vi "Efficiency+LLR.vi"() -> ()   [LabVIEW 2020]
doc: "Demonstrates how to use triggers and events to synchronize multiple channels in Sequence source mode. Use this example to sequence multiple channels in lock-step."
uses:
  controls/eff_llr_nightwing_config.ctl
  controls/eff_llr_heatwave_config.ctl
  pmbus_ltm4676a/controls/ltm4676a_config.ctl
  controls/eff_llr_system_timing_config.ctl
  <instrlib>/niDCPower/nidcpower.llb/niDCPower Sense.ctl
  <instrlib>/niDCPower/nidcpower.llb/niDCPower Wait For Event - Event.ctl
  <instrlib>/niDCPower/nidcpower.llb/niDCPower Source Mode.ctl
  <instrlib>/niDCPower/nidcpower.llb/niDCPower Output Function.ctl
  <instrlib>/niDCPower/nidcpower.llb/niDCPower Sequence Attribute Type.ctl
  <vilib>/Analysis/1siggen.llb/Ramp Pattern by Samples.vi
  <instrlib>/niDCPower/nidcpower.llb/niDCPower Create Advanced Sequence Step.vi
  <instrlib>/niDCPower/nidcpower.llb/niDCPower Configure Digital Edge Source Trigger.vi
  <instrlib>/niDCPower/nidcpower.llb/niDCPower Configure Digital Edge Measure Trigger.vi
  <vilib>/Utility/file.llb/Write Delimited Spreadsheet (string).vi
  <vilib>/Utility/file.llb/Write Delimited Spreadsheet (DBL).vi
  <vilib>/Analysis/NI_AALBase.lvlib
panel:
  in  "App control":enum32{"Main", "Info", "Ref", "Debug"}(tab)
  out "Test time (s)":dbl
  in  "Config control":T1(tab)
  in  "Source config":T2={"Source device name"="PXIe-4151", "Source device channel"="0", "Source current limit (A)"=25.0, "Source power boundary (W)"=300.0, "Source values (V)"=[9.0, 12.0, 18.0, 20.0]}
  in  "Load config":T3={"Load device name"="PXIe-4051", "Load device channel"="0", "Load voltage limit (V)"=6.0, "Sweep type"=1, "Points or Points/Decade"=10, "Current load level start"=0.1, "Current load level stop"=24.0} {"Current load level stop" min=0.0 step=0.1; "Current load level start" min=0.0 step=0.1; "Points or Points/Decade" min=1; "Sweep type" items=["Linear", "Logarithmic"]}
  in  "System timing config":T4={"DUT setup time (s)"=1.0, "Source delay (s)"=0.005, "Aperture time (s)"=0.005, "Timeout (s)"=15.0} {"Timeout (s)" format="%.3p"; "DUT setup time (s)" format="%.2p"}
  in  "LTM4676A Runtime Config":T5={"SDC config path"=path "C:/dev/users/qkocian/opp_support/demos/argus-buck-demo/instrumentstudio/sdc/pmbus_ltm4676a.sdconfig", "Output setpoint (V)"=3.3, "Voltage margin (%)"=5.0, "Voltage warn limit (%)"=7.5, "Voltage fault limit (%)"=10.0, "Switching frequency (kHz)"=650} {"Switching frequency (kHz)" items=["250"=62440, "350"=64188, "425"=64338, "500"=64488, "575"=575, "650"=650, "750"=750, "1000"=1000]; "Voltage fault limit (%)" min=0.0 max=100.0 step=1.0 format="%.1g"; "Voltage warn limit (%)" min=0.0 max=100.0 step=1.0 format="%.1g"; "Voltage margin (%)" min=0.0 max=100.0 step=1.0 format="%.1g"; "Output setpoint (V)" min=0.5 max=5.5 step=0.1}
  out "Load Current (A) vs DUT Output Voltage (V)":T6(graph) caption="Current (Amps) vs Voltage (Volts)"
  out "DUT Efficiency (%) vs. Load Current (A)":cluster{dbl[], dbl[]}[](graph) caption="Current (Amps) vs Voltage (Volts)"
  in  "Use PMBus?":bool
  out "success?":bool
  in  "Export debug curves?":enum16{"No", "Yes"}(ring)
  out "Load Power":T7(graph) caption="Current (Amps) vs Voltage (Volts)"
  out "Supply Power":T7(graph) caption="Current (Amps) vs Voltage (Volts)"
  out "Load Current":T7(graph) caption="Current (Amps) vs Voltage (Volts)"
  out "Load Voltage":cluster{dbl[], "voltage measurements":dbl[]}(graph) caption="Current (Amps) vs Voltage (Volts)"
  out "Supply Current":T7(graph) caption="Current (Amps) vs Voltage (Volts)"
  out "Supply Voltage":T8(graph) caption="Current (Amps) vs Voltage (Volts)"
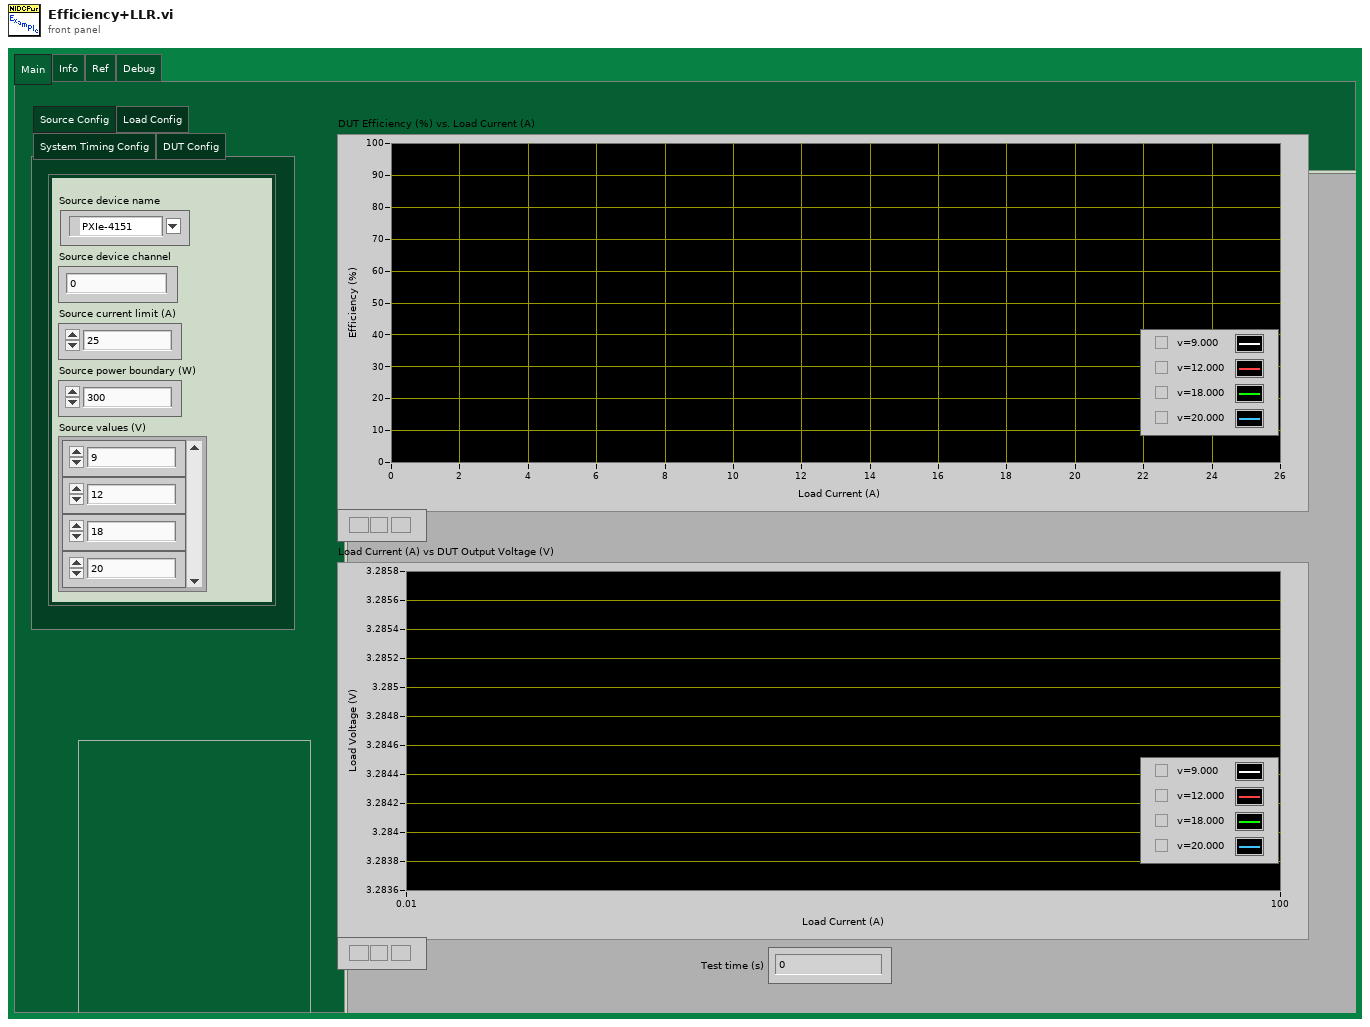
[diagram p1: front panel]
types:
  T1 = enum32{"Source Config", "Load Config", "System Timing Config", "DUT Config"}
  T2 = typedef "eff_llr_nightwing_config.ctl" = cluster{"Source device name":refnum<k15>, "Source device channel":string, "Source current limit (A)":dbl, "Source power boundary (W)":dbl, "Source values (V)":dbl[]}
  T3 = typedef "eff_llr_heatwave_config.ctl" = cluster{"Load device name":refnum<k15>, "Load device channel":string, "Load voltage limit (V)":dbl, "Sweep type":u16, "Points or Points/Decade":i32, "Current load level start":dbl, "Current load level stop":dbl}
  T4 = typedef "eff_llr_system_timing_config.ctl" = cluster{"DUT setup time (s)":dbl, "Source delay (s)":dbl, "Aperture time (s)":dbl, "Timeout (s)":dbl}
  T5 = typedef "ltm4676a_config.ctl" = cluster{"SDC config path":path, "Output setpoint (V)":dbl, "Voltage margin (%)":dbl, "Voltage warn limit (%)":dbl, "Voltage fault limit (%)":dbl, "Switching frequency (kHz)":u16}
  T6 = cluster{"current measurements":dbl[], "voltage measurements":dbl[]}[]
  T7 = cluster{"Ramp Pattern":dbl[], "current measurements":dbl[]}
  T8 = cluster{"Ramp Pattern":dbl[], "voltage measurements":dbl[]}
  T9 = typedef "niDCPower Source Mode.ctl" = i32
  T10 = typedef "niDCPower Wait For Event - Event.ctl" = i32
  T11 = typedef "niDCPower Sense.ctl" = i32
  T12 = typedef "niDCPower Sequence Attribute Type.ctl" = i32
  T13 = typedef "niDCPower Output Function.ctl" = i32
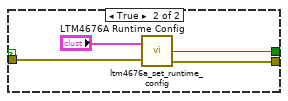
[diagram p2: hidden frame]
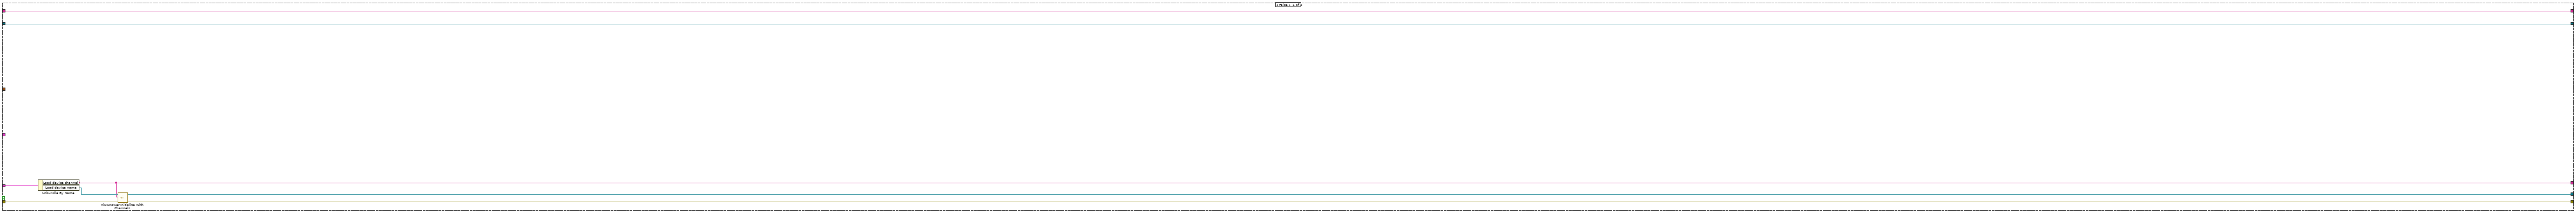
[diagram p3: hidden frame]
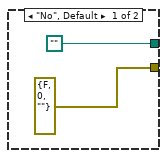
[diagram p5: hidden frame]
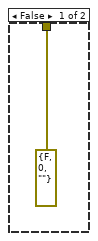
[diagram p6: hidden frame]
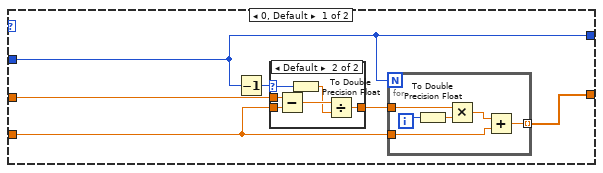
[diagram p7: hidden frame]
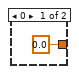
[diagram p8: hidden frame]
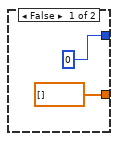
[diagram p9: hidden frame]
diagram:
  w25 = 1038 items=["Slow"=1041, "Normal"=1038, "Fast"=1039, "Custom"=1042] ("Source:Transient Response")
  w35 = T9 1020 items=["Single Point"=1020, "Sequence"=1021] ("source mode")
  w40 = 1006 items=["DC Voltage"=1006, "DC Current"=1007, "Pulse Voltage"=1049, "Pulse Current"=1050] ("Source:Output Function")
  w47 = T10 1030 items=["Source Complete Event"=1030, "Measure Complete Event"=1031, "Sequence Iteration Complete Event"=1032, "Sequence Engine Done Event"=1033, "Pulse Complete Event"=1051, "Ready For Pulse Trigger Event"=1052] ("event")
  w50 = 1 items=["Off", "On"] ("Source:DC Current:Current Level Autorange")
  w53 = T11 1009 items=["Local"=1008, "Remote"=1009] ("sense")
  n1 = Unbundle By Name("Source config") -> ("Source device channel"=w14:string, "Source device name"=w18:refnum<k15>)
  n2 = call <instrlib>:"niDCPower Initialize With Channels.vi"("channels"=w14, "resource name"=w18) -> ("error out"=w51:errorcluster, "instrument handle out"=w52:refnum<k15>)  [unwired: 3 in, 5 out]
  n3 = Unbundle By Name("System timing config") -> ("DUT setup time (s)"=w20:dbl)
  n4 = Unbundle By Name("Source config") -> ("Source values (V)"=w15:dbl[], "Source current limit (A)"=w17:dbl)
  n5 = call <instrlib>:"niDCPower Configure Sense.vi"("error in (no error)"=w51, "sense"=w53, "channel name"=w14, "instrument handle"=w52) -> ("error out"=w37:errorcluster, "instrument handle out"=w39:refnum<k15>)  [unwired: 6 in]
  n6 = call <instrlib>:"niDCPower Configure Source Mode With Channels.vi"("error in (no error)"=w37, "source mode"=w35, "channel name"=w14, "instrument handle"=w39) -> ("error out"=w36:errorcluster, "instrument handle out"=w38:refnum<k15>)  [unwired: 6 in]
  n7 = Index Array(array=w15, index=0) -> (element=w42:dbl)
  n8 = property class="niDCPower"(reference=w38, error in=w36, "Active Channel"=w14, "Output Function"=w40, "Voltage Level"=w42, "Current Limit"=w17, "Voltage Level Autorange"=w50, "Current Limit Autorange"=w50, "Source Delay"=w20) -> (reference out=w27:refnum<k15>, error out=w26:errorcluster)
  n9 = property class="niDCPower"(reference=w27, error in=w26, "Active Channel"=w14, "Transient Response"=w25) -> (reference out=w23:refnum<k15>, error out=w24:errorcluster)
  n10 = call <instrlib>:"niDCPower Commit With Channels.vi"("error in (no error)"=w24, "channel name"=w14, "instrument handle"=w23) -> ("error out"=w21:errorcluster, "instrument handle out"=w22:refnum<k15>)  [unwired: 7 in]
  n11 = call <instrlib>:"niDCPower Initiate With Channels.vi"("error in (no error)"=w21, "channel name"=w14, "instrument handle"=w22) -> ("error out"=w49:errorcluster, "instrument handle out"=w48:refnum<k15>)  [unwired: 7 in]
  n12 = call <instrlib>:"niDCPower Wait For Event With Channels.vi"("error in (no error)"=w49, "event"=w47, "channel name"=w14, "instrument handle"=w48) -> ("error out"=w46:errorcluster, "instrument handle out"=w45:refnum<k15>)  [unwired: 6 in]
  n13 = call <instrlib>:"niDCPower Measure Multiple.vi"("error in (no error)"=w46, "channel name"=w14, "instrument handle"=w45) -> ("error out"=w43:errorcluster, "instrument handle out"=w44:refnum<k15>)  [unwired: 5 in, 2 out]
  n14 = call <instrlib>:"niDCPower Abort With Channels.vi"("error in (no error)"=w43, "channel name"=w14, "instrument handle"=w44) -> ("error out"=w13:errorcluster, "instrument handle out"=w41:refnum<k15>)  [unwired: 7 in]
  n15 = case shown="False" "Use PMBus?" {
    tunnel: w13 -> [w59 w63]
    tunnel: [w59 w61] -> w12
    tunnel: [TRUE ("success?") w60] -> w4
    frame False {
    }
    frame True {
      n16 = call "ltm4676a_set_runtime_config.vi"("LTM4676A Runtime Config"="LTM4676A Runtime Config", "error in (no error)"=w63) -> ("success?"=w60:bool, "error out"=w61:errorcluster)  [unwired: 1 out]
    }
  }
  "success?" <- w4
  n17 = call <vilib>:"High Resolution Relative Seconds.vi"() -> ("relative seconds"=w2:dbl)
  n18 = case shown="True" w4 {
    tunnel: w41 -> [w68 w141]
    tunnel: [w64 w129] -> w28
    tunnel: "System timing config" -> [_ w104]
    tunnel: "Source config" -> [_ w98]
    tunnel: w14 -> [w69 w94]
    tunnel: w12 -> [w66 w88]
    tunnel: [w66 w84] -> w9
    tunnel: [w68 w83] -> w7
    tunnel: [w69 w82] -> w6
    tunnel: [w65 w81] -> w5
    tunnel: "Load config" -> [w67 w73]
    tunnel: w2 -> [_ w72]
    frame False {
      n19 = Unbundle By Name(w67) -> ("Load device channel"=w64:string, "Load device name"=w65:refnum<k15>)
      n20 = call <instrlib>:"niDCPower Initialize With Channels.vi"("error in (no error)"=w66, "channels"=w64, "resource name"=w65) -> ()  [unwired: 2 in, 7 out]
    }
    frame True {
      w119 = 1038 items=["Slow"=1041, "Normal"=1038, "Fast"=1039, "Custom"=1042] ("Source:Transient Response")
      w131 = T9 1020 items=["Single Point"=1020, "Sequence"=1021] ("source mode")
      w148 = T10 1030 items=["Source Complete Event"=1030, "Measure Complete Event"=1031, "Sequence Iteration Complete Event"=1032, "Sequence Engine Done Event"=1033, "Pulse Complete Event"=1051, "Ready For Pulse Trigger Event"=1052] ("event")
      w153 = 1 items=["Off", "On"] ("Source:DC Current:Current Level Autorange")
      w154 = 1007 items=["DC Voltage"=1006, "DC Current"=1007, "Pulse Voltage"=1049, "Pulse Current"=1050] ("Source:Output Function")
      w173 = T11 1009 items=["Local"=1008, "Remote"=1009] ("sense")
      w178 = 1 items=["Off", "On"] ("DC Voltage:Voltage Level Autorange")
      w179 = T12[] [1250001, 1250005] items=["Source -> Output Function"=1150008, "Source -> Output Enabled"=1250006, "Source -> Output Resistance"=1150061, "Source -> Transient Response"=1150062, "Source -> Custom Transient Response -> Voltage Gain Bandwidth"=1150067, "Source -> Custom Transient Response -> Voltage Compensation Frequency"=1150068, "Source -> Custom Transient Response -> Voltage Pole-Zero Ratio"=1150069, "Source -> Custom Transient Response -> Current Gain Bandwidth"=1150070, "Source -> Custom Transient Response -> Current Compensation Frequency"=1150071, "Source -> Custom Transient Response -> Current Pole-Zero Ratio"=1150072, "Source -> DC Voltage -> Voltage Level"=1250001, "Source -> DC Voltage -> Voltage Level Range"=1150005, "Source -> DC Voltage -> Current Limit"=1250005, "Source -> DC Voltage -> Current Limit High"=1150187, "Source -> DC Voltage -> Current Limit Low"=1150188, "Source -> DC Voltage -> Current Limit Range"=1150004, "Source -> DC Current -> Current Level"=1150009, "Source -> DC Current -> Current Level Range"=1150011, "Source -> DC Current -> Voltage Limit"=1150010, "Source -> DC Current -> Voltage Limit High"=1150185, "Source -> DC Current -> Voltage Limit Low"=1150186, "Source -> DC Current -> Voltage Limit Range"=1150012, "Source -> Pulse Voltage -> Pulse Voltage Level"=1150080, "Source -> Pulse Voltage -> Pulse Bias Voltage Level"=1150082, "Source -> Pulse Voltage -> Pulse Voltage Level Range"=1150084, "Source -> Pulse Voltage -> Pulse Current Limit"=1150081, "Source -> Pulse Voltage -> Pulse Current Limit High"=1150193, "Source -> Pulse Voltage -> Pulse Current Limit Low"=1150194, "Source -> Pulse Voltage -> Pulse Bias Current Limit"=1150083, "Source -> Pulse Voltage -> Pulse Bias Current Limit High"=1150195, "Source -> Pulse Voltage -> Pulse Bias Current Limit Low"=1150196, "Source -> Pulse Voltage -> Pulse Current Limit Range"=1150085, "Source -> Pulse Current -> Pulse Current Level"=1150086, "Source -> Pulse Current -> Pulse Bias Current Level"=1150088, "Source -> Pulse Current -> Pulse Current Level Range"=1150090, "Source -> Pulse Current -> Pulse Voltage Limit"=1150087, "Source -> Pulse Current -> Pulse Voltage Limit High"=1150189, "Source -> Pulse Current -> Pulse Voltage Limit Low"=1150190, "Source -> Pulse Current -> Pulse Bias Voltage Limit"=1150089, "Source -> Pulse Current -> Pulse Bias Voltage Limit High"=1150191, "Source -> Pulse Current -> Pulse Bias Voltage Limit Low"=1150192, "Source -> Pulse Current -> Pulse Voltage Limit Range"=1150091, "Source -> Advanced -> Source Delay"=1150051, "Source -> Advanced -> Pulse Bias Delay"=1150092, "Source -> Advanced -> Pulse On Time"=1150093, "Source -> Advanced -> Pulse Off Time"=1150094, "Source -> Advanced -> OVP Enabled"=1250002, "Source -> Advanced -> OVP Limit"=1250003, "Source -> Advanced -> Compliance Limit Symmetry"=1150184, "Source -> Advanced -> Sequence Step Delta Time"=1150198, "Measurement -> Sense"=1150013, "Measurement -> Aperture Time"=1150058, "Measurement -> Measure Record Length"=1150063, "Measurement -> Advanced -> DC Noise Rejection"=1150066, "Measurement -> Autorange"=1150244, "Measurement -> Advanced -> Autorange Behavior"=1150245, "Measurement -> Advanced -> Autorange Aperture Time Mode"=1150246, "Measurement -> Advanced -> Autorange Minimum Aperture Time"=1150247, "Measurement -> Advanced -> Autorange Minimum Aperture Time Units"=1150248, "Measurement -> Advanced -> Autorange Minimum Current Range"=1150255, "Measurement -> Advanced -> Autorange Minimum Voltage Range"=1150256, "Measurement -> Advanced -> Autorange Threshold Mode"=1150257, "Measurement -> Advanced -> Autorange Maximum Delay After Range Change"=1150322, "LCR -> Instrument Mode"=1150208, "LCR -> LCR Stimulus Function"=1150209, "LCR -> LCR Frequency"=1150210, "LCR -> LCR Voltage Amplitude"=1150211, "LCR -> LCR Current Amplitude"=1150212, "LCR -> LCR DC Bias Source"=1150213, "LCR -> LCR DC Bias Voltage Level"=1150214, "LCR -> LCR DC Bias Current Level"=1150215, "LCR -> LCR Impedance Autorange"=1150216, "LCR -> LCR Impedance Range"=1150217, "LCR -> LCR Measurement Time"=1150218, "LCR -> LCR Custom Measurement Time"=1150258, "LCR -> LCR Source Delay Mode"=1150315, "LCR -> Compensation -> Open -> Enabled"=1150220, "LCR -> Compensation -> Open -> Conductance"=1150261, "LCR -> Compensation -> Open -> Susceptance"=1150262, "LCR -> Compensation -> Short -> Enabled"=1150221, "LCR -> Compensation -> Short -> Resistance"=1150263, "LCR -> Compensation -> Short -> Reactance"=1150264, "LCR -> Compensation -> Load -> Enabled"=1150222, "LCR -> Compensation -> Load -> Measured Resistance"=1150268, "LCR -> Compensation -> Load -> Measured Reactance"=1150269, "LCR -> Compensation -> Load -> Actual Resistance"=1150270, "LCR -> Compensation -> Load -> Actual Reactance"=1150271] ("advanced sequence properties")
      w112 = "SourceVoltages" ("sequence name")
      w182 = T13 1007 items=["DC Voltage"=1006, "DC Current"=1007, "Pulse Voltage"=1049, "Pulse Current"=1050] ("output function")
      w183 = 1027 items=["Automatically after Source Complete"=1025, "On Demand"=1026, "On Measure Trigger"=1027] ("Measurement:Advanced:Measure When")
      w184 = T9 1021 items=["Single Point"=1020, "Sequence"=1021] ("source mode")
      w191 = T13 1006 items=["DC Voltage"=1006, "DC Current"=1007, "Pulse Voltage"=1049, "Pulse Current"=1050] ("output function")
      w128 = 1025 items=["Automatically after Source Complete"=1025, "On Demand"=1026, "On Measure Trigger"=1027] ("Measurement:Advanced:Measure When")
      w198 = T9 1021 items=["Single Point"=1020, "Sequence"=1021] ("source mode")
      n21 = Unbundle By Name(w73) -> ("Load device channel"=w75:string, "Load device name"=w74:refnum<k15>)
      n22 = Unbundle By Name(w73) -> ("Load voltage limit (V)"=w80:dbl, "Sweep type"=w79:u16, "Points or Points/Decade"=w78:i32, "Current load level stop"=w77:dbl, "Current load level start"=w76:dbl)
      n23 = local read "System timing config"() -> (w109:T4)
      n24 = call <instrlib>:"niDCPower Initialize With Channels.vi"("error in (no error)"=w88, "channels"=w75, "resource name"=w74) -> ("error out"=w151:errorcluster, "instrument handle out"=w152:refnum<k15>)  [unwired: 2 in, 5 out]
      n25 = Unbundle By Name(w109) -> ("DUT setup time (s)"=w108:dbl)
      n26 = call <instrlib>:"niDCPower Configure Sense.vi"("error in (no error)"=w151, "sense"=w173, "channel name"=w75, "instrument handle"=w152) -> ("error out"=w134:errorcluster, "instrument handle out"=w135:refnum<k15>)  [unwired: 6 in]
      n27 = call <instrlib>:"niDCPower Configure Source Mode With Channels.vi"("error in (no error)"=w134, "source mode"=w131, "channel name"=w75, "instrument handle"=w135) -> ("error out"=w132:errorcluster, "instrument handle out"=w133:refnum<k15>)  [unwired: 6 in]
      n28 = case shown="1" w79 {
        tunnel: w78 -> [w327 w346]
        tunnel: [w330 w350] -> w175
        tunnel: w76 -> [w329 w347]
        tunnel: w77 -> [w328 w354]
        tunnel: [w327 w351] -> w168
        frame 0, Default {
          n29 = Decrement(x=w327) -> (x-1=w332:i32)
          n30 = case shown="Default" w332 {
            selector: w332 -> [_ w340]
            tunnel: w328 -> [_ w345]
            tunnel: w329 -> [_ w344]
            tunnel: [0.0 w342] -> w331
            frame 0 {
            }
            frame Default {
              n31 = Subtract(x=w345, y=w344) -> (x-y=w343:dbl)
              n32 = To Double Precision Float(number=w340) -> (double precision float=w341:dbl)
              n33 = Divide(x=w343, y=w341) -> (x/y=w342:dbl)
            }
          }
          n34 = for {
            N: w327 -> [_]
            tunnel: w331 -> [w337]
            tunnel: w329 -> [w338]
            tunnel: [w333] -> w330 mode=indexing
            i -> [w336]
            n35 = To Double Precision Float(number=w336) -> (double precision float=w334:dbl)
            n36 = Multiply(x=w337, y=w334) -> (x*y=w335:dbl)
            n37 = Add(x=w335, y=w338) -> (x+y=w333:dbl)
          }
        }
        frame 1 {
          n38 = Divide(x=w354, y=w347) -> (x/y=w355:dbl)
          n39 = Logarithm Base 10(1:w355) -> (0:w352:dbl)
          n40 = In Range and Coerce(upper limit=inf, x=w352, lower limit=0.0) -> (In Range?=w349:bool)  [unwired: 1 out]
          n41 = case shown="True" w349 {
            tunnel: [dbl[] [] w365] -> w350
            tunnel: [0 w358] -> w351
            tunnel: w354 -> [_ w364]
            tunnel: w347 -> [_ w363]
            tunnel: w346 -> [_ w360]
            frame False {
            }
            frame True {
              n42 = Reciprocal(x=w360) -> (1/x=w362:dbl)
              n43 = Power Of 10(x=w362) -> (10^x=w361:dbl)
              n44 = while {
                tunnel: w361 -> [w370]
                tunnel: w363 -> [w373]
                tunnel: [w369] -> w365 mode=indexing
                tunnel: [w371] -> w359
                tunnel: w364 -> [w366]
                i -> [w371]
                stop <- w368 continue-if-true
                n45 = Power Of X(1:w370, 2:w371) -> (0:w372:dbl)
                n46 = Multiply(x=w372, y=w373) -> (x*y=w367:dbl)
                n47 = Less?(x=w367, y=w366) -> (x < y?=w368:bool)
                n48 = Select(t=w367, s=w368, f=w366) -> (s? t:f=w369:dbl)
              }
              n49 = Increment(x=w359) -> (x+1=w358:i32)
            }
          }
        }
      }
      n50 = property class="niDCPower"(reference=w133, error in=w132, "Active Channel"=w75, "Output Function"=w154, "Current Level"=1.0 ("Source:DC Current:Current Level"), "Voltage Limit Range"=w80, "Current Level Autorange"=w153, "Source Delay"=w108, "Current Level Range"=40.0 ("Source:DC Current:Current Level Range")) -> (reference out=w121:refnum<k15>, error out=w120:errorcluster)
      n51 = property class="niDCPower"(reference=w121, error in=w120, "Active Channel"=w75, "Transient Response"=w119) -> (reference out=w116:refnum<k15>, error out=w115:errorcluster)
      n52 = Multiply(x=w175, y=1.0) -> (x*y=w163:dbl[])
      n53 = local read "Source config"() -> (w103:T2)
      n54 = call <instrlib>:"niDCPower Commit With Channels.vi"("error in (no error)"=w115, "channel name"=w75, "instrument handle"=w116) -> ("error out"=w118:errorcluster, "instrument handle out"=w117:refnum<k15>)  [unwired: 7 in]
      n55 = call <instrlib>:"niDCPower Initiate With Channels.vi"("error in (no error)"=w118, "channel name"=w75, "instrument handle"=w117) -> ("error out"=w150:errorcluster, "instrument handle out"=w149:refnum<k15>)  [unwired: 7 in]
      n56 = Unbundle By Name(w103) -> ("Source values (V)"=w102:dbl[])
      n57 = call <instrlib>:"niDCPower Wait For Event With Channels.vi"("error in (no error)"=w150, "event"=w148, "channel name"=w75, "instrument handle"=w149) -> ("error out"=w147:errorcluster, "instrument handle out"=w146:refnum<k15>)  [unwired: 6 in]
      n58 = call <instrlib>:"niDCPower Measure Multiple.vi"("error in (no error)"=w147, "channel name"=w75, "instrument handle"=w146) -> ("error out"=w144:errorcluster, "instrument handle out"=w145:refnum<k15>)  [unwired: 5 in, 2 out]
      n59 = Array Size(array=w102) -> (size(s)=w110:i32)
      n60 = call <instrlib>:"niDCPower Abort With Channels.vi"("error in (no error)"=w144, "channel name"=w75, "instrument handle"=w145) -> ("error out"=w139:errorcluster, "instrument handle out"=w140:refnum<k15>)  [unwired: 7 in]
      n61 = for {
        N: w110 -> [_]
        tunnel: w163 -> [w246]
        tunnel: [w245] -> w162 mode=concatenating
        n62 = for {
          tunnel: w246 -> [w247] mode=indexing
          tunnel: [w247] -> w245 mode=indexing
        }
      }
      n63 = call <instrlib>:"niDCPower Configure Source Mode.vi"("error in (no error)"=w139, "source mode"=w198, "instrument handle"=w141) -> ("error out"=w200:errorcluster, "instrument handle out"=w199:refnum<k15>)  [unwired: 7 out]
      n64 = call <instrlib>:"niDCPower Configure Output Function.vi"("error in (no error)"=w200, "output function"=w191, "channel name"=w94, "instrument handle"=w199) -> ("error out"=w142:errorcluster, "instrument handle out"=w143:refnum<k15>)  [unwired: 6 out]
      n65 = property class="niDCPower"(reference=w143, error in=w142, "Active Channel"=w94, "Source:DC Voltage:Voltage Level Autorange"=w178, "Source:DC Voltage:Current Limit Autorange"=w178) -> (reference out=w177:refnum<k15>, error out=w176:errorcluster)
      n66 = Unbundle By Name(w104) -> ("Source delay (s)"=w107:dbl)
      n67 = property class="niDCPower"(reference=w177, error in=w176, "Active Channel"=w94, "Source Delay"=w107) -> (reference out=w91:refnum<k15>, error out=w90:errorcluster)
      n68 = Unbundle By Name(w98) -> ("Source power boundary (W)"=w101:dbl, "Source values (V)"=w100:dbl[], "Source current limit (A)"=w99:dbl)
      n69 = call <instrlib>:"niDCPower Create Advanced Sequence.vi"("instrument handle"=w91, "sequence name"=w112, "advanced sequence properties"=w179, "error in (no error)"=w90) -> ("instrument handle out"=w181:refnum<k15>, "error out"=w180:errorcluster)  [unwired: 10 in]
      n70 = for {
        tunnel: w101 -> [w377]
        tunnel: w99 -> [w376]
        tunnel: w100 -> [w375] mode=indexing
        shift-right: [w379] -> w96
        shift-left: w181 -> [w381]
        shift-right: [w378] -> w95
        shift-left: w180 -> [w380]
        tunnel: w168 -> [w374]
        n71 = for {
          N: w374 -> [_]
          shift-right: [w390] -> w378
          shift-left: w380 -> [w393]
          shift-right: [w389] -> w379
          shift-left: w381 -> [w388]
          tunnel: w377 -> [w387]
          tunnel: w375 -> [w382]
          tunnel: w376 -> [w385]
          n72 = call-poly <instrlib>:"niDCPower Create Advanced Sequence Step (Poly).vi"("error in (no error)"=w393, "instrument handle"=w388) -> ("error out"=w391:errorcluster, "instrument handle out"=w392:refnum<k15>)  [unwired: 8 in]
          n73 = Divide(x=w387, y=w382) -> (x/y=w384:dbl)
          n74 = Less?(x=w384, y=w385) -> (x < y?=w386:bool)
          n75 = Select(t=w384, s=w386, f=w385) -> (s? t:f=w383:dbl)
          n76 = property class="niDCPower"(reference=w392, error in=w391, "Voltage Level"=w382, "Current Limit"=w383) -> (reference out=w389:refnum<k15>, error out=w390:errorcluster)
        }
      }
      n77 = call "buildTerminalName.vi"("error in (no error)"=w95, "Local Terminal Name"="SourceTrigger", "Channel Name"=w94, "session handle"=w96) -> ("error IO"=w92:errorcluster, "Fully Qualified Terminal Name"=w194:string, "session handle 2"=w93:refnum<k15>)  [unwired: 5 out]
      n78 = call "buildTerminalName.vi"("error in (no error)"=w92, "Local Terminal Name"="SourceCompleteEvent", "Channel Name"=w94, "session handle"=w93) -> ("error IO"=w111:errorcluster, "Fully Qualified Terminal Name"=w193:string, "session handle 2"=w127:refnum<k15>)  [unwired: 5 out]
      n79 = Unbundle By Name(w104) -> ("Aperture time (s)"=w106:dbl)
      n80 = property class="niDCPower"(reference=w127, error in=w111, "Measure When"=w128, "Aperture Time"=w106) -> (reference out=w197:refnum<k15>, error out=w196:errorcluster)
      n81 = call <instrlib>:"niDCPower Commit.vi"("error in (no error)"=w196, "instrument handle"=w197) -> ("error out"=w138:errorcluster, "instrument handle out"=w159:refnum<k15>)  [unwired: 8 out]
      n82 = call <instrlib>:"niDCPower Configure Source Mode.vi"("error in (no error)"=w138, "source mode"=w184, "instrument handle"=w140) -> ("error out"=w186:errorcluster, "instrument handle out"=w185:refnum<k15>)  [unwired: 7 out]
      n83 = call <instrlib>:"niDCPower Configure Output Function.vi"("error in (no error)"=w186, "output function"=w182, "instrument handle"=w185) -> ("error out"=w136:errorcluster, "instrument handle out"=w137:refnum<k15>)  [unwired: 1 in, 6 out]
      n84 = call <instrlib>:"niDCPower Set Sequence.vi"("error in (no error)"=w136, "values"=w162, "instrument handle"=w137) -> ("error out"=w164:errorcluster, "instrument handle out"=w165:refnum<k15>)  [unwired: 2 in, 5 out]
      n85 = disable-structure shown="Disabled" {
        disable-tunnel: [w214 w217] -> w172
        disable-tunnel: [w213 w216] -> w171
        disable-tunnel: w165 -> [w212 w217]
        disable-tunnel: w164 -> [w211 w216]
        disable-tunnel: w75 -> [w210 _]
        frame Disabled {
          w215 = 1 items=["Off", "On"] ("DC Voltage:Voltage Level Autorange")
          n86 = property class="niDCPower"(reference=w212, error in=w211, "Active Channel"=w210, "Current Level Autorange"=w215) -> (reference out=w214:refnum<k15>, error out=w213:errorcluster)
        }
        frame Enabled {
        }
      }
      n87 = property class="niDCPower"(reference=w172, error in=w171, "Active Channel"=w75, "Source Delay"=0.0 ("Source:Advanced:Source Delay")) -> (reference out=w167:refnum<k15>, error out=w166:errorcluster)
      n88 = call-poly <instrlib>:"niDCPower Configure Trigger (Poly).vi"("error in (no error)"=w166, "input terminal"=w194, "instrument handle"=w167) -> ("error out"=w189:errorcluster, "instrument handle out"=w190:refnum<k15>)  [unwired: 1 in, 6 out]
      n89 = Unbundle By Name(w104) -> ("Timeout (s)"=w89:dbl, "Aperture time (s)"=w105:dbl)
      n90 = property class="niDCPower"(reference=w190, error in=w189, "Measure When"=w183, "Aperture Time"=w105) -> (reference out=w187:refnum<k15>, error out=w188:errorcluster)
      n91 = call-poly <instrlib>:"niDCPower Configure Trigger (Poly).vi"("error in (no error)"=w188, "input terminal"=w193, "instrument handle"=w187) -> ("error out"=w161:errorcluster, "instrument handle out"=w160:refnum<k15>)  [unwired: 1 in, 6 out]
      n92 = call <instrlib>:"niDCPower Commit.vi"("error in (no error)"=w161, "instrument handle"=w160) -> ("error out"=w201:errorcluster, "instrument handle out"=w202:refnum<k15>)  [unwired: 8 out]
      n93 = flat-sequence {
        tunnel: w202 -> [w225]
        tunnel: w201 -> [w224]
        tunnel: w159 -> [w221]
        tunnel: [w222] -> w209
        tunnel: [w220] -> w208
        tunnel: [w219] -> w207
        tunnel: w89 -> [w218]
        tunnel: [w218] -> w206
        tunnel: w209 -> [w232]
        tunnel: w208 -> [w230]
        tunnel: w207 -> [w227]
        tunnel: [w232] -> w205
        tunnel: [w228] -> w204
        tunnel: [w229] -> w203
        tunnel: w206 -> [w226]
        tunnel: [w234] -> w123
        tunnel: [w235] -> w122
        tunnel: [w236] -> w170
        tunnel: w205 -> [w236]
        tunnel: w204 -> [w235]
        tunnel: w203 -> [w234]
        tunnel: [w233] -> w113
        frame #0 {
          n94 = call <instrlib>:"niDCPower Initiate.vi"("error in (no error)"=w224, "instrument handle"=w225) -> ("error out"=w223:errorcluster, "instrument handle out"=w219:refnum<k15>)  [unwired: 8 out]
          n95 = call <instrlib>:"niDCPower Initiate.vi"("error in (no error)"=w223, "instrument handle"=w221) -> ("error out"=w220:errorcluster, "instrument handle out"=w222:refnum<k15>)  [unwired: 8 out]
        }
        frame #1 {
          w231 = T10 1033 items=["Source Complete Event"=1030, "Measure Complete Event"=1031, "Sequence Iteration Complete Event"=1032, "Sequence Engine Done Event"=1033] ("event")
          n96 = call <instrlib>:"niDCPower Wait For Event.vi"("timeout (10.0)"=w226, "error in (no error)"=w230, "event"=w231, "instrument handle"=w227) -> ("error out"=w228:errorcluster, "instrument handle out"=w229:refnum<k15>)  [unwired: 6 out]
        }
        frame #2 {
          n97 = call <vilib>:"High Resolution Relative Seconds.vi"() -> ("relative seconds"=w233:dbl)
        }
      }
      n98 = case shown="\"Yes\"" "Export debug curves?" {
        tunnel: [errorcluster {"status"=FALSE, "code"=0, "source"=""} ("error out") w240] -> w157
        tunnel: [path "" w239] -> w156
        frame "No", Default {
        }
        frame "Yes" {
          n99 = Format Date/Time String(time format string (%c)="export\\%Y%m%d_%H%M%S") -> (date/time string=w241:string)  [unwired: 2 in]
          n100 = call <vilib>:"Application Directory.vi"() -> ("Application Directory"=w242:path)
          n101 = Build Path(base path=w242, name or relative path=w241) -> (appended path=w243:path)
          n102 = Create Folder(path (use dialog)=w243) -> (created path=w239:path, error out=w240:errorcluster)  [unwired: 2 in, 1 out]
        }
      }
      n103 = Unbundle By Name(w98) -> ("Source values (V)"=w97:dbl[])
      n104 = Subtract(x=w113, y=w72) -> (x-y=→"Test time (s)":dbl)
      n105 = for {
        tunnel: w75 -> [w299]
        tunnel: w94 -> [w298]
        shift-right: [w301] -> w155
        shift-left: w123 -> [w282]
        shift-right: [w300] -> w130
        shift-left: w122 -> [w281]
        shift-right: [w302] -> w169
        shift-left: w170 -> [w303]
        tunnel: w168 -> [w254]
        tunnel: w97 -> [w250] mode=indexing
        tunnel: w157 -> [w270]
        tunnel: w156 -> [w269]
        tunnel: [w299] -> w129
        tunnel: [w298] -> w82
        tunnel: [w273] -> w126 mode=indexing
        tunnel: [w272] -> w125 mode=indexing
        i -> [w274]
        # "Debug curves"
        # "Main sequence; Retrieve data"
        # "Main plot legend"
        n106 = call <vilib>:"Check if File or Folder Exists.vi"("error in (no error)"=w270, "path"=w269) -> ("error out"=w267:errorcluster, "file or folder exists?"=w271:bool, "dup path"=w268:path)  [unwired: 7 in]
        n107 = call <instrlib>:"niDCPower Fetch Multiple.vi"("instrument handle"=w303, "channel name"=w298, "count (1)"=w254, "error in (no error)"=w281) -> ("instrument handle out"=w302:refnum<k15>, "voltage measurements"=w259:dbl[], "current measurements"=w258:dbl[], "error out"=w297:errorcluster)  [unwired: 1 in, 7 out]
        n108 = call-poly <vilib>:"Ramp Pattern.vi"("start"=1.0, "end"=w254, "samples"=w254) -> ("Ramp Pattern"=w253:dbl[])  [unwired: 7 in, 1 out]
        n109 = call <instrlib>:"niDCPower Fetch Multiple.vi"("instrument handle"=w282, "channel name"=w299, "count (1)"=w254, "error in (no error)"=w297) -> ("instrument handle out"=w301:refnum<k15>, "voltage measurements"=w256:dbl[], "current measurements"=w248:dbl[], "error out"=w285:errorcluster)  [unwired: 1 in, 7 out]
        n110 = Multiply "Load power (W)"(x=w256, y=w248) -> (x*y=w289:dbl[])
        n111 = Multiply "Source power (W)"(x=w259, y=w258) -> (x*y=w288:dbl[])
        n112 = To Unsigned Long Integer(number=w274) -> (unsigned 32bit integer=w278:u32)
        n113 = To Unsigned Long Integer(number=w274) -> (unsigned 32bit integer=w293:u32)
        n114 = Absolute Value "Load currents"(x=w248) -> (abs(x)=w290:dbl[])
        n115 = Absolute Value(x=w289) -> (abs(x)=w255:dbl[])
        n116 = Absolute Value(x=w288) -> (abs(x)=w257:dbl[])
        n117 = Format Value(format string="%.3f", value (0)=w250) -> (output string=w277:string)  [unwired: 1 out]
        n118 = Format Value(format string="%.3f", value (0)=w250) -> (output string=w294:string)  [unwired: 1 out]
        n119 = Increment(x=w278) -> (x+1=w279:u32)
        n120 = Increment(x=w293) -> (x+1=w292:u32)
        n121 = Divide(x=w255, y=w257) -> (x/y=w287:dbl[])
        n122 = Concatenate Strings(" v=" ("string"), w277) -> (w251:string)
        n123 = Absolute Value "Load currents"(x=w248) -> (abs(x)=w249:dbl[])
        n124 = Concatenate Strings(" v=" ("string"), w294) -> (w252:string)
        n125 = property on="Load Current (A) vs DUT Output Voltage (V)" class="XYGraph (strict)"("LegNumRows"=w279) -> (error out=w280:errorcluster)  [unwired: 2 in, 1 out]
        n126 = property on="DUT Efficiency (%) vs. Load Current (A)" class="XYGraph (strict)"("LegNumRows"=w292) -> (error out=w291:errorcluster)  [unwired: 2 in, 1 out]
        n127 = Multiply "Efficiency (%)"(x=w287, y=100.0) -> (x*y=w283:dbl[])
        n128 = case shown="True" w271 {
          tunnel: w250 -> [_ w326]
          tunnel: w267 -> [_ w325]
          tunnel: w268 -> [_ w324]
          tunnel: [errorcluster {"status"=FALSE, "code"=0, "source"=""} ("error out") w323] -> w284
          tunnel: w259 -> [_ w322]
          tunnel: w258 -> [_ w321]
          tunnel: w256 -> [_ w320]
          tunnel: w248 -> [_ w319]
          tunnel: w283 -> [_ w318]
          tunnel: w257 -> [_ w306]
          tunnel: w255 -> [_ w305]
          frame False {
          }
          frame True {
            w309 = "," ("delimiter (\\t)")
            # "Test data export"
            n129 = Format Value(format string="efficiency_vsource_%.2fV.csv" ("string"), value (0)=w326) -> (output string=w316:string)  [unwired: 1 out]
            n130 = Build Path(base path=w324, name or relative path=w316) -> (appended path=w315:path)
            n131 = call-poly <vilib>:"Write Delimited Spreadsheet.vi"("file path (dialog if empty)"=w315, "2D data"=string[][] [["Supply voltage (V)", "Supply current (A)", "Supply power (W)", "Load voltage (V)", "Load current (A)", "Load power (W)", "Efficiency (%)"]], "error in (no error)"=w325, "delimiter (\\t)"=w309) -> ("new file path (Not A Path if cancelled)"=w313:path, "error out"=w312:errorcluster)  [unwired: 10 in]
            n132 = Build Array(w322, w321, w306, w320, w319, w305, w318) -> (w310:dbl[][])
            n133 = call-poly <vilib>:"Write Delimited Spreadsheet.vi"("file path (dialog if empty)"=w313, "format (%.3f)"="%.6f", "2D data"=w310, "append to file? (new file:F)"=TRUE, "error in (no error)"=w312, "transpose? (no:F)"=TRUE, "delimiter (\\t)"=w309) -> ("error out"=w323:errorcluster)  [unwired: 7 in, 1 out]
          }
        }
        n134 = property on="Load Current (A) vs DUT Output Voltage (V)" class="XYGraph (strict)"(error in=w280, "Active Plot"=w278, "Plot.Plot Name"=w251) -> ()  [unwired: 1 in, 2 out]
        n135 = property on="DUT Efficiency (%) vs. Load Current (A)" class="XYGraph (strict)"(error in=w291, "Active Plot"=w293, "Plot.Plot Name"=w252) -> ()  [unwired: 1 in, 2 out]
        n136 = Bundle(w249, "voltage measurements"=w256) -> (w272:cluster{dbl[], "voltage measurements":dbl[]})  [unwired: 1 out]
        n137 = Bundle(w290, w283) -> (w273:cluster{dbl[], dbl[]})  [unwired: 1 out]
        n138 = Merge Errors(w285, w284) -> (w300:errorcluster)
        n139 = Bundle("Ramp Pattern"=w253, "voltage measurements"=w259) -> (→"Supply Voltage":T8)  [unwired: 1 out]
        n140 = Bundle("Ramp Pattern"=w253, "current measurements"=w258) -> (→"Supply Current":T7)  [unwired: 1 out]
        n141 = Bundle("Ramp Pattern"=w253, w257) -> (→"Supply Power":cluster{"Ramp Pattern":dbl[], dbl[]})  [unwired: 1 out]
        n142 = Bundle("Ramp Pattern"=w253, "voltage measurements"=w256) -> (→"Load Voltage":T8)  [unwired: 1 out]
        n143 = Bundle("Ramp Pattern"=w253, "current measurements"=w248) -> (→"Load Current":T7)  [unwired: 1 out]
        n144 = Bundle("Ramp Pattern"=w253, w255) -> (→"Load Power":cluster{"Ramp Pattern":dbl[], dbl[]})  [unwired: 1 out]
      }
      "DUT Efficiency (%) vs. Load Current (A)" <- w126
      "Load Current (A) vs DUT Output Voltage (V)" <- w125
      n145 = call <instrlib>:"niDCPower Abort With Channels.vi"("error in (no error)"=w130, "channel name"=w129, "instrument handle"=w155) -> ("error out"=w87:errorcluster, "instrument handle out"=w81:refnum<k15>)  [unwired: 7 in]
      n146 = call <instrlib>:"niDCPower Abort With Channels.vi"("error in (no error)"=w87, "channel name"=w82, "instrument handle"=w169) -> ("error out"=w85:errorcluster, "instrument handle out"=w86:refnum<k15>)  [unwired: 7 in]
      n147 = call <instrlib>:"niDCPower Delete Advanced Sequence With Channels.vi"("error in (no error)"=w85, "sequence name"=w112, "channel name"=w82, "instrument handle"=w86) -> ("error out"=w84:errorcluster, "instrument handle out"=w83:refnum<k15>)  [unwired: 6 in]
    }
  }
  n148 = call <instrlib>:"niDCPower Configure Output Enabled.vi"("error in (no error)"=w9, "output enabled"=FALSE, "channel name"=w28, "instrument handle"=w5) -> ("error out"=w31:errorcluster, "instrument handle out"=w32:refnum<k15>)  [unwired: 6 in]
  n149 = call <instrlib>:"niDCPower Reset With Channels.vi"("error in (no error)"=w31, "channel name"=w28, "instrument handle"=w32) -> ("error out"=w57:errorcluster, "instrument handle out"=w56:refnum<k15>)  [unwired: 7 in]
  n150 = call <instrlib>:"niDCPower Close.vi"("error in (no error)"=w57, "instrument handle"=w56) -> ("error out"=w8:errorcluster)  [unwired: 9 out]
  n151 = call <instrlib>:"niDCPower Configure Output Enabled.vi"("error in (no error)"=w8, "output enabled"=FALSE, "channel name"=w6, "instrument handle"=w7) -> ("error out"=w10:errorcluster, "instrument handle out"=w11:refnum<k15>)  [unwired: 6 in]
  n152 = call <instrlib>:"niDCPower Reset With Channels.vi"("error in (no error)"=w10, "channel name"=w6, "instrument handle"=w11) -> ("error out"=w54:errorcluster, "instrument handle out"=w55:refnum<k15>)  [unwired: 7 in]
  n153 = call <instrlib>:"niDCPower Close.vi"("error in (no error)"=w54, "instrument handle"=w55) -> ("error out"=w30:errorcluster)  [unwired: 9 out]
  n154 = call <vilib>:"Simple Error Handler.vi"("error in (no error)"=w30) -> ()  [unwired: 1 in, 8 out]
